vi "APX VarianTMP AP2.vi"() -> ()   [LabVIEW 2015]
uses:
  <vilib>/Instr/_visa.llb/VISA Configure Serial Port (Instr).vi
  <userlib>/caLab/Private/Get_PV-1D.vi
  <userlib>/caLab/Private/Put_DBL-1D_PV-1D.vi
  <userlib>/caLab/Private/Put_DBL_PV.vi
panel:
  out "APX:AP2TruboS":dbl
  out "TMPC5STRSTP 2":string
  out "APX:AP2Trubo_STOP":bool
  out "APX:AP2Turbo_START":bool
  out "TMPC5STRSTP":string
  out "SERIAL":string
  out "V-501":refnum<visa-resource-name>="COM4"
  out "APX:AP2TurboF":dbl caption="F_20/Hz"
  out "APX:AP2TurboP":dbl caption="P_20/W"
  out "APX:AP2TurboS:STR":string
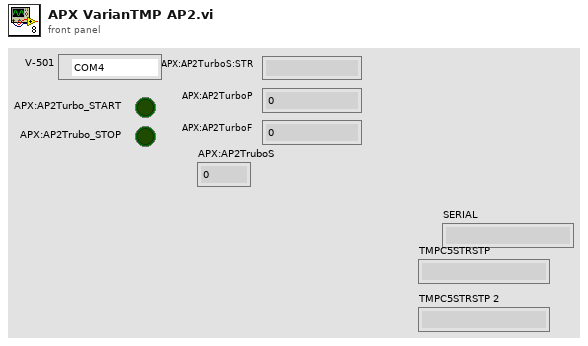
[diagram p1: front panel]
types:
  T1 = enum16{"START", "STOP", "REMOTE/SERIAL", "REMOTE", "SERIAL", "START/STOP", "PUMP STATUS", "Driving Frequency", "PUMP POWER", "PRESSURE"}
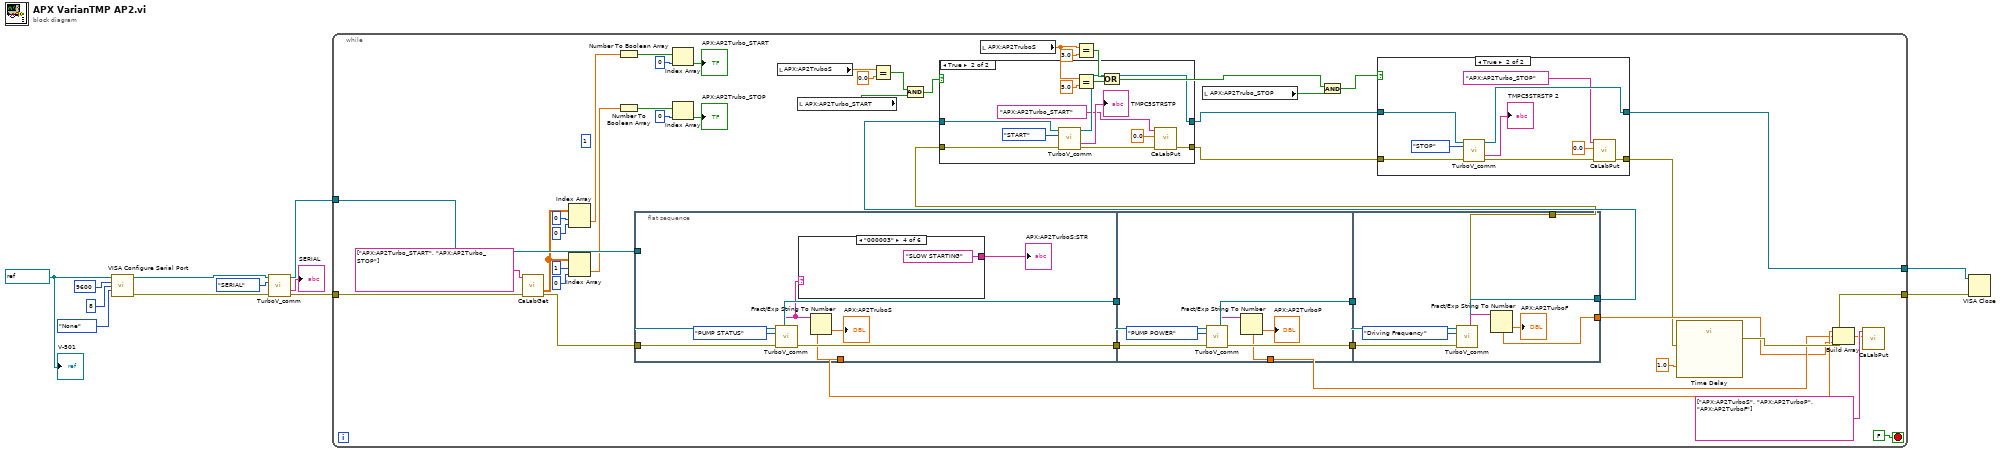
[diagram p0: block diagram]
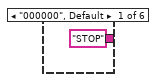
[diagram p2: hidden frame]
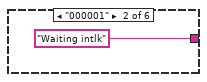
[diagram p3: hidden frame]
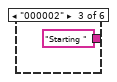
[diagram p4: hidden frame]
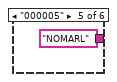
[diagram p5: hidden frame]
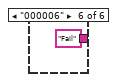
[diagram p6: hidden frame]
diagram:
  w12 = refnum<visa-resource-name> "COM6" ("VISA resource name")
  n1 = call-poly "VISA Configure Serial Port"("VISA resource name"=w12, "baud rate (9600)"=u32 9600, "data bits (8)"=u16 8, "parity (0:none)"=enum16{"None", "Odd", "Even", "Mark", "Space"}."None") -> ("VISA resource name out"=w5:refnum<visa-resource-name>, "error out"=w3:errorcluster)  [unwired: 10 in]
  n2 = call "TurboV_comm.vi"("VISA resource name"=w5, "Command"=T1."SERIAL", "error in (no error)"=w3) -> ("VISA resource name out"=w4:refnum<visa-resource-name>, "read buffer"=→"SERIAL":string, "error out"=w2:errorcluster)  [unwired: 10 in]
  n3 = while {
    tunnel: w4 -> [w60]
    tunnel: w2 -> [w40]
    tunnel: [w14] -> w8
    tunnel: [w58] -> w7
    stop <- FALSE stop-if-true
    (unwired) 1
    n4 = call-poly "CaLabGet.vi"("PV Names"=string[] ["APX:AP2Turbo_START", "APX:AP2Turbo_STOP"], "Error in (no error)"=w40) -> ("Value Array (number)"=w41:dbl[][], "Error out"=w39:errorcluster)  [unwired: 7 in, 5 out]
    n5 = Index Array(array=w41, index (row)=0 ("disabled index (row)"), index (col)=0 ("index (row)")) -> (element=w47:dbl)
    n6 = Index Array(array=w41, index (row)=1 ("disabled index (row)"), index (col)=0 ("index (row)")) -> (element=w42:dbl)
    n7 = Number To Boolean Array(number=w47) -> (Boolean array=w49:bool[])
    n8 = Number To Boolean Array(number=w42) -> (Boolean array=w44:bool[])
    n9 = flat-sequence {
      tunnel: w60 -> [w68]
      tunnel: w39 -> [w67]
      tunnel: [w66] -> w29
      tunnel: [w65] -> w28
      tunnel: [w61] -> w56
      tunnel: w29 -> [w80]
      tunnel: w28 -> [w77]
      tunnel: [w79] -> w27
      tunnel: [w78] -> w26
      tunnel: [w75] -> w55
      tunnel: w27 -> [w88]
      tunnel: w26 -> [w87]
      tunnel: [w84] -> w24
      tunnel: [w83] -> w54
      tunnel: [w82] -> w23
      frame #0 {
        n10 = call "TurboV_comm.vi"("VISA resource name"=w68, "Command"=T1."PUMP STATUS", "error in (no error)"=w67) -> ("VISA resource name out"=w66:refnum<visa-resource-name>, "read buffer"=w62:string, "error out"=w65:errorcluster)  [unwired: 10 in]
        n11 = case shown="\"000003\"" w62 {
          tunnel: ["STOP" "Waiting intlk" "Starting " "SLOW STARTING" "NOMARL" "Fail"] -> w63
          frame "000000", Default {
          }
          frame "000001" {
          }
          frame "000002" {
          }
          frame "000003" {
          }
          frame "000005" {
          }
          frame "000006" {
          }
        }
        "APX:AP2TurboS:STR" <- w63
        n12 = Fract/Exp String To Number(string=w62) -> (number=w61:dbl)  [unwired: 3 in, 1 out]
        "APX:AP2TruboS" <- w61
      }
      frame #1 {
        n13 = call "TurboV_comm.vi"("VISA resource name"=w80, "Command"=T1."PUMP POWER", "error in (no error)"=w77) -> ("VISA resource name out"=w79:refnum<visa-resource-name>, "read buffer"=w76:string, "error out"=w78:errorcluster)  [unwired: 10 in]
        n14 = Fract/Exp String To Number(string=w76) -> (number=w75:dbl)  [unwired: 3 in, 1 out]
        "APX:AP2TurboP" <- w75
      }
      frame #2 {
        n15 = call "TurboV_comm.vi"("VISA resource name"=w88, "Command"=T1."Driving Frequency", "error in (no error)"=w87) -> ("VISA resource name out"=w84:refnum<visa-resource-name>, "read buffer"=w85:string, "error out"=w82:errorcluster)  [unwired: 10 in]
        n16 = Fract/Exp String To Number(string=w85) -> (number=w83:dbl)  [unwired: 3 in, 1 out]
        "APX:AP2TurboF" <- w83
      }
    }
    n17 = Index Array(array=w49, index=0) -> (element=→"APX:AP2Turbo_START":bool)
    n18 = Index Array(array=w44, index=0) -> (element=→"APX:AP2Trubo_STOP":bool)
    n19 = local read "APX:AP2TruboS"() -> (w30:dbl)
    n20 = local read "APX:AP2Turbo_START"() -> (w18:bool)
    n21 = Equal?(x=w30, y=0.0) -> (x = y?=w20:bool)
    n22 = And(x=w20, y=w18) -> (x .and. y?=w19:bool)
    n23 = case shown="True" w19 {
      tunnel: [w90 w97] -> w22
      tunnel: [w89 w91] -> w21
      tunnel: w24 -> [w90 w96]
      tunnel: w23 -> [w89 w95]
      frame False {
      }
      frame True {
        n24 = call "TurboV_comm.vi"("VISA resource name"=w96, "Command"=T1."START", "error in (no error)"=w95) -> ("VISA resource name out"=w97:refnum<visa-resource-name>, "read buffer"=→"TMPC5STRSTP":string, "error out"=w92:errorcluster)  [unwired: 10 in]
        n25 = call-poly <userlib>:"CaLabPut.vi"("Error in (no error)"=w92, "Value"=0.0, "PV Name"="APX:AP2Turbo_START") -> ("Error out"=w91:errorcluster)  [unwired: 5 in, 3 out]
      }
    }
    n26 = local read "APX:AP2TruboS"() -> (w36:dbl)
    n27 = Equal?(x=w36, y=3.0) -> (x = y?=w34:bool)
    n28 = Equal?(x=w36, y=5.0) -> (x = y?=w35:bool)
    n29 = Or(x=w34, y=w35) -> (x .or. y?=w17:bool)
    n30 = local read "APX:AP2Trubo_STOP"() -> (w15:bool)
    n31 = And(x=w17, y=w15) -> (x .and. y?=w16:bool)
    n32 = case shown="True" w16 {
      tunnel: [w101 w109] -> w14
      tunnel: [w100 w102] -> w13
      tunnel: w22 -> [w101 w108]
      tunnel: w21 -> [w100 w107]
      frame False {
      }
      frame True {
        n33 = call "TurboV_comm.vi"("VISA resource name"=w108, "Command"=T1."STOP", "error in (no error)"=w107) -> ("VISA resource name out"=w109:refnum<visa-resource-name>, "read buffer"=→"TMPC5STRSTP 2":string, "error out"=w103:errorcluster)  [unwired: 10 in]
        n34 = call-poly <userlib>:"CaLabPut.vi"("Error in (no error)"=w103, "Value"=0.0, "PV Name"="APX:AP2Turbo_STOP") -> ("Error out"=w102:errorcluster)  [unwired: 5 in, 3 out]
      }
    }
    n35 = call "Time Delay"("error in (no error)"=w13, "Delay Time (s)"=1.0) -> ("error out"=w58:errorcluster)  [unwired: 9 in]
    n36 = Build Array(w56, w55, w54) -> (w53:dbl[])
    n37 = call-poly <userlib>:"CaLabPut.vi"("Values"=w53, "PV Names"=string[] ["APX:AP2TurboS", "APX:AP2TurboP", "APX:AP2TurboF"]) -> ()  [unwired: 6 in, 4 out]
  }
  n38 = VISA Close(VISA resource name=w8, error in (no error)=w7) -> ()  [unwired: 1 out]
  "V-501" <- w12
